vi "CreateControlTerminals.vi"(8 "error in":errorcluster, 11 "PythonConverter_BD in":refnum<class "PyConvBD.lvclass">) -> (0 "error out":errorcluster, 3 "PythonConverter_BD out":refnum<class "PyConvBD.lvclass">)   [LabVIEW 2014, in "Raspberry Pi Compatible Compiler for LabVIEW.lvlib" / "PyConvBD.lvclass"]
uses:
  PyConvBD.lvclass
  PyConvBD.lvclass/PyConvBD.ctl
  VI Interpreter/Classes/ControlTerminal/ControlTerminal.lvclass
  VI Interpreter/Classes/VI Interpreter/VI Interpreter.lvclass
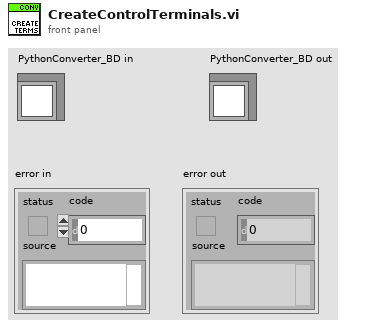
[diagram p1: front panel]
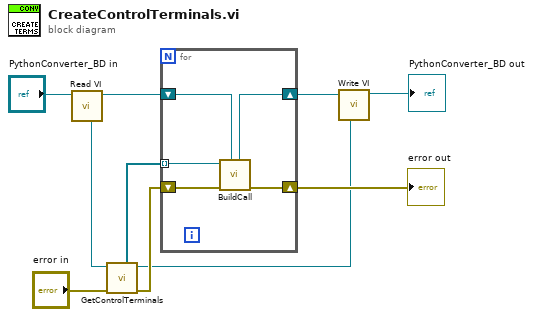
[diagram p0: block diagram]
diagram:
  n1 = call "Read VI.vi"("PythonConverter_BD in"="PythonConverter_BD in") -> ("PythonConverter_BD out"=w6:refnum<class "PyConvBD.lvclass">, "VI Interpreter"=w5:refnum<class "VI Interpreter.lvclass">)  [unwired: 7 in]
  n2 = call "GetControlTerminals.vi"("error in"="error in", "VI Interpreter in"=w5) -> ("error out"=w9:errorcluster, "VI Interpreter out"=w2:refnum<class "VI Interpreter.lvclass">, "controls"=w8:refnum<class "ControlTerminal.lvclass">[])  [unwired: 5 in]
  n3 = for {
    tunnel: w8 -> [w14] mode=indexing
    shift-right: [w11] -> w10
    shift-left: w9 -> [w15]
    shift-right: [w12] -> w3
    shift-left: w6 -> [w13]
    n4 = call-dynamic "BuildCall.vi"("PythonConverter_BD in"=w13, "error in"=w15, "Control Terminal in"=w14) -> ("error out"=w11:errorcluster, "PythonConverter_BD out"=w12:refnum<class "PyConvBD.lvclass">)  [unwired: 6 in, 1 out]
  }
  "error out" <- w10
  n5 = call "Write VI.vi"("VI Interpreter"=w2, "PythonConverter_BD in"=w3) -> ("PythonConverter_BD out"=→"PythonConverter_BD out":refnum<class "PyConvBD.lvclass">)  [unwired: 7 in]
